vi "colArrayToCommaString.vi"(1 "array":string[](array[string])) -> (0 "comma string":string)   [LabVIEW 2019, in "libpqutility.lvlib"]
doc: "converts a string array into comma separeted string"
uses:
  libpqutility.lvlib
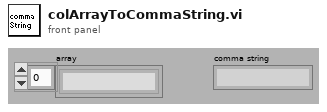
[diagram p1: front panel]
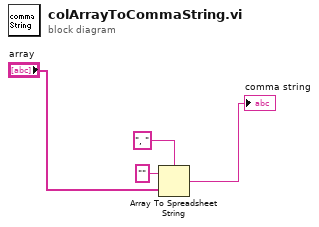
[diagram p0: block diagram]
diagram:
  n1 = Array To Spreadsheet String(delimiter (Tab)=", " ("Trennzeichen (Tab)"), array="array", 3:"" ("Format-String")) -> (spreadsheet string=→"comma string":string)
